vi "Filter Class Tree_by Label_3.vi"(6 "Show":T1={"Show Private"=TRUE, "Show Scripting"=FALSE}, 10 "Filter Str":string, 11 "Class Tree Array":T2[](array[typedef])) -> (3 "Class Tree Array":T2[](array[typedef]))   [LabVIEW 2023]
uses:
  class/Class Item Cluster.ctl
  <userlib>/_OpenG.lib/array/array.llb/Filter 1D Array with Scalar (I32)__ogtk.vi
  <userlib>/_OpenG.lib/array/array.llb/Index 1D Array Elements (Variant)__ogtk.vi
  <userlib>/_OpenG.lib/array/array.llb/Remove Duplicates from 1D Array (I32)__ogtk.vi
panel:
  out "Out size":i32
  out "In Size":i32
  # "To maintain tree indents, we must retain all parents (as disabled) if they don't match the filter, or else the tree item inset will break"
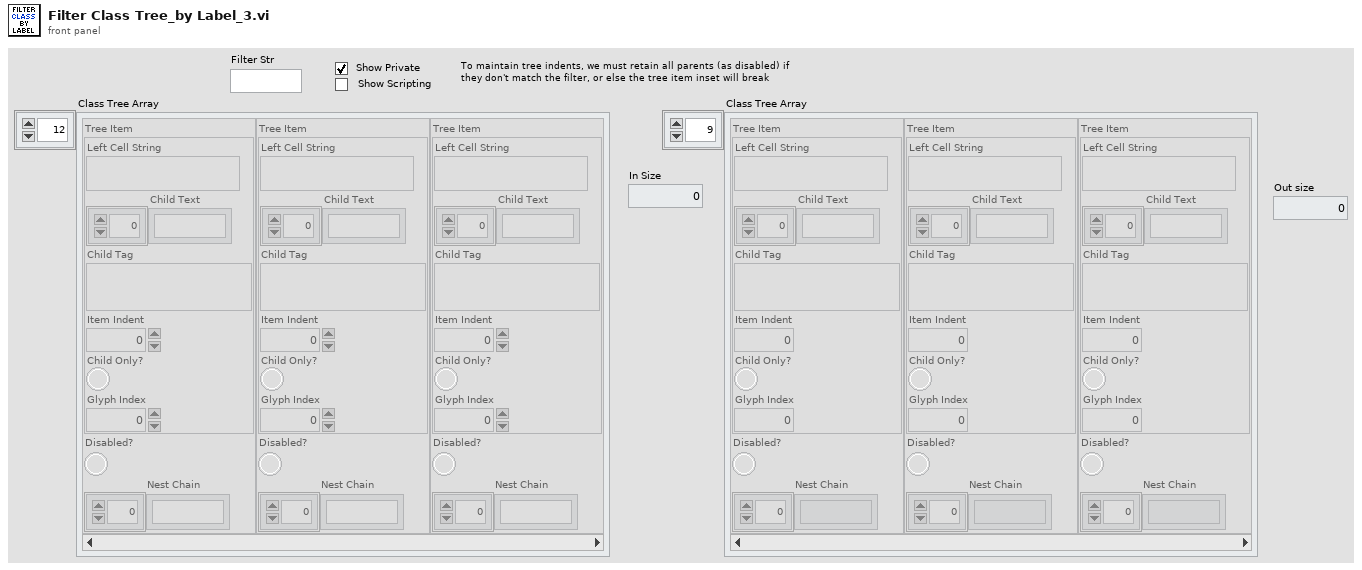
[diagram p1: front panel]
types:
  T1 = cluster{"Show Private":bool, "Show Scripting":bool}
  T2 = typedef "Class Item Cluster.ctl" = cluster{"Tree Item":cluster{"Left Cell String":string, "Child Text":string[], "Child Tag":string, "Item Indent":i32, "Child Only?":bool, "Glyph Index":i32}, "Disabled?":bool, "Nest Chain":string[]}
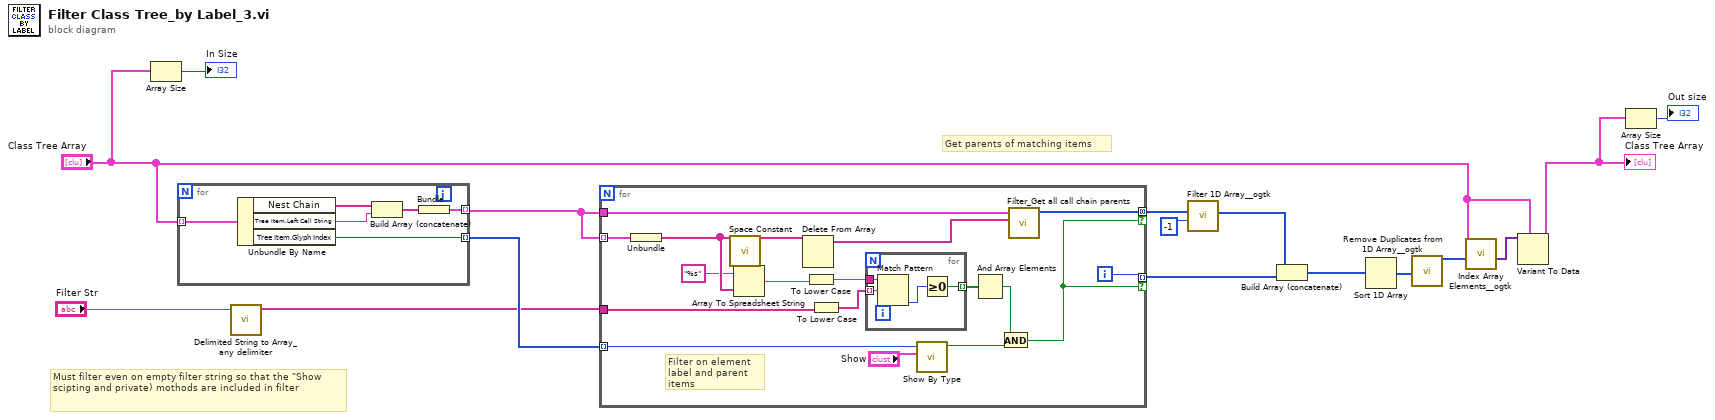
[diagram p0: block diagram]
diagram:
  # "Must filter even on empty filter string so that the \"Show scipting and private) mothods are included in filter"
  # "Get parents of matching items"
  n1 = Array Size(array="Class Tree Array") -> (size(s)=→"In Size":i32)
  n2 = for {
    tunnel: "Class Tree Array" -> [w22] mode=indexing
    tunnel: [w18] -> w12 mode=indexing
    tunnel: [w17] -> w5 mode=indexing
    n3 = Unbundle By Name(w22) -> ("Nest Chain"=w21:string[], "Tree Item.Left Cell String"=w20:string, "Tree Item.Glyph Index"=w17:i32)
    n4 = Build Array (concatenate)(w21, w20) -> (w19:string[])
    n5 = Bundle(w19) -> (w18:cluster{string[]})  [unwired: 1 in]
  }
  n6 = call "Delimited String to Array_any delimiter.vi"("Delimted String"="Filter Str") -> ("Array"=w3:string[])  [unwired: 10 in]
  n7 = for {
    tunnel: w12 -> [w30] mode=indexing
    tunnel: w12 -> [w39]
    tunnel: [w40] -> w11 mode=indexing if=w26
    tunnel: [w38] -> w9 mode=concatenating if=w26
    tunnel: w3 -> [w35]
    tunnel: w5 -> [w25] mode=indexing
    i -> [w40]
    # "Filter on element label and parent items"
    n8 = Unbundle(w30) -> (w34:string[])
    n9 = call <vilib>:"Space Constant.vi"() -> ("String"=w32:string)
    n10 = Array To Spreadsheet String(delimiter (Tab)=w32, array=w34, 3:"%s" ("format string")) -> (spreadsheet string=w31:string)
    n11 = Delete From Array(array=w34) -> (array with subset deleted=w24:string[])  [unwired: 2 in, 1 out]
    n12 = To Lower Case(string=w31) -> (all lower case string=w37:string)
    n13 = To Lower Case(string=w35) -> (all lower case string=w36:string[])
    n14 = for {
      tunnel: w37 -> [w43]
      tunnel: w36 -> [w42] mode=indexing
      tunnel: [w41] -> w27 mode=indexing
      n15 = Match Pattern(string=w43, regular expression=w42) -> (offset past match=w44:i32)  [unwired: 1 in, 3 out]
      n16 = Greater Or Equal To 0?(x=w44) -> (x >= 0?=w41:bool)
    }
    n17 = call "Show By Type.vi"("Show"="Show", "Item's Property Type"=w25) -> ("Show"=w28:bool)  [unwired: 9 in]
    n18 = And Array Elements(Boolean array=w27) -> (logical AND=w23:bool)
    n19 = And(x=w23, y=w28) -> (x .and. y?=w26:bool)
    n20 = call "Filter_Get all call chain parents.vi"("Call Chain"=w24, "Array"=w39) -> ("parent indicies"=w38:i32[])  [unwired: 9 in]
  }
  n21 = call-poly <userlib>:"Filter 1D Array__ogtk.vi"("items to filter"=-1, "array"=w9) -> ("filtered array"=w7:i32[])  [unwired: 4 in, 1 out]
  n22 = Build Array (concatenate)(w7, w11) -> (w10:i32[])
  n23 = Sort 1D Array(array=w10) -> (sorted array=w2:i32[])
  n24 = call-poly <userlib>:"Remove Duplicates from 1D Array__ogtk.vi"("Input Array"=w2) -> ("Output Array"=w1:i32[])  [unwired: 1 out]
  n25 = call-poly <userlib>:"Index Array Elements__ogtk.vi"("indices"=w1, "array"="Class Tree Array") -> ("elements"=w6:variant[])  [unwired: 9 in]
  n26 = Variant To Data(type="Class Tree Array", Variant=w6) -> (data=w14:T2[])  [unwired: 1 in, 1 out]
  "Class Tree Array" <- w14
  n27 = Array Size(array=w14) -> (size(s)=→"Out size":i32)
